vi "ToScale.vi"(8 "error in":errorcluster, 11 "Scale in":refnum<class "Generic.lvclass">) -> (0 "error out":errorcluster, 3 "Scale out":refnum<class "Scale.lvclass">)   [LabVIEW 2014, in "Raspberry Pi Compatible Compiler for LabVIEW.lvlib" / "Scale.lvclass"]
uses:
  Scale.lvclass
  Generic/Generic.lvclass
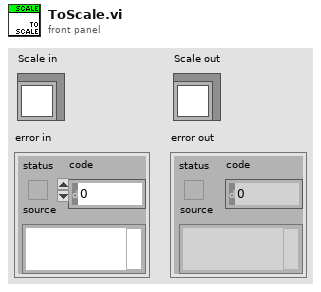
[diagram p1: front panel]
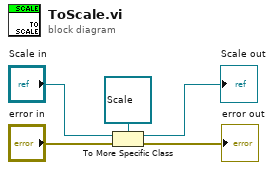
[diagram p0: block diagram]
diagram:
  n1 = To More Specific Class(target class=refnum<class "Scale.lvclass"> refnum ("Scale.lvclass"), reference="Scale in", error in="error in") -> (specific class reference=→"Scale out":refnum<class "Scale.lvclass">, error out=→"error out":errorcluster)
